vi "Side Pane Width and Height.vi"(8 "error in (no error)":errorcluster) -> (0 "error out":errorcluster, 2 "Width":dbl, 3 "Height":dbl)   [LabVIEW 2014]
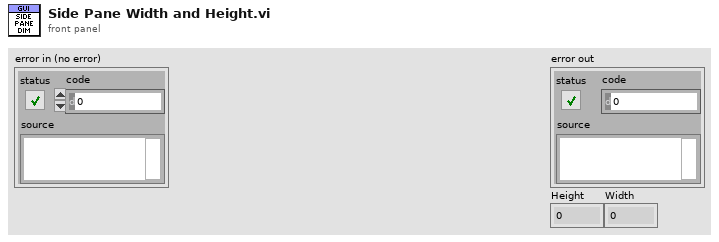
[diagram p1: front panel]
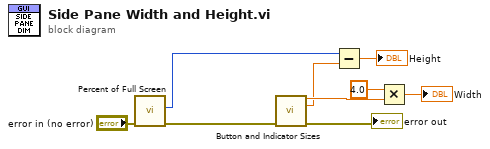
[diagram p0: block diagram]
diagram:
  n1 = call "Percent of Full Screen.vi"("error in (no error)"="error in (no error)") -> ("error out"=w5:errorcluster, "Bottom"=w7:i16)  [unwired: 8 in, 1 out]
  n2 = call "Button and Indicator Sizes.vi"("error in (no error)"=w5) -> ("Button Width"=w9:dbl, "Button Height"=w6:dbl, "error out"=→"error out":errorcluster)  [unwired: 10 in, 2 out]
  n3 = Subtract(x=w7, y=w6) -> (x-y=→"Height":dbl)
  n4 = Multiply(x=4.0, y=w9) -> (x*y=→"Width":dbl)
